vi "Create Channels From Line Name.vi"(11 "String":string) -> (1 "channel":refnum<class "TBM channel.lvclass">, 2 "channel 2":refnum<class "TBM channel.lvclass">, 3 "TBM channel out":refnum<class "TBM channel.lvclass">)   [LabVIEW 2018, in "Benchmark PID configuration.lvclass"]
uses:
  Benchmark PID configuration.lvclass
  <vilib>/NI/Tag Bus Module Framework/channel/TBM channel.lvclass
  <vilib>/NI/Tag Bus Module Framework/channel/channel classification.ctl
  <vilib>/NI/Tag Bus/tag/Data Type.ctl
  <vilib>/NI/Tag Bus/tag/tag descriptor.lvclass
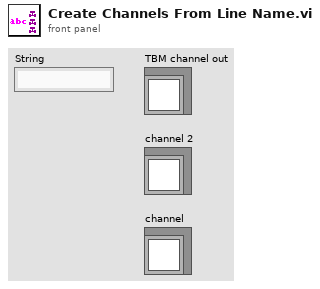
[diagram p1: front panel]
types:
  T1 = typedef "TBM channel.lvclass/channel classification.ctl" = enum16{"input data", "output data", "processing parameter", "processing result"}
  T2 = typedef "tag bus.lvlib/tag descriptor.lvclass/Data Type.ctl" = enum16{"Double", "Single", "I64", "I32", "I16", "I8", "U64", "U32", "U16", "U8", "Boolean", "String", "Array of Double", "Array of Single", "Array of I64", "Array of I32", "Array of I16", "Array of I8", "Array of U64", "Array of U32", "Array of U16", "Array of U8", "Array of Boolean", "Array of String"}
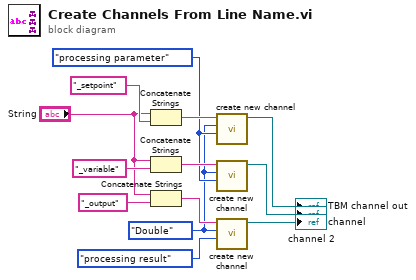
[diagram p0: block diagram]
diagram:
  w4 = Data_Type."Double" ("data type")
  w5 = channel_classification."processing parameter" ("channel classification")
  n1 = Concatenate Strings("String", "_setpoint" ("string")) -> (w11:string)
  n2 = Concatenate Strings("String", "_variable" ("string")) -> (w12:string)
  n3 = Concatenate Strings("String", "_output" ("string")) -> (w13:string)
  n4 = call <vilib>:"create new channel.vi"("channel classification"=w5, "data type"=w4, "channel name"=w11) -> ("channel"=→"TBM channel out":refnum<class "TBM channel.lvclass">)  [unwired: 8 in]
  n5 = call <vilib>:"create new channel.vi"("channel classification"=w5, "data type"=w4, "channel name"=w12) -> ("channel"=→"channel 2":refnum<class "TBM channel.lvclass">)  [unwired: 8 in]
  n6 = call <vilib>:"create new channel.vi"("channel classification"=channel_classification."processing result", "data type"=w4, "channel name"=w13) -> ("channel"=→"channel":refnum<class "TBM channel.lvclass">)  [unwired: 8 in]
